vi "LED Main Loop.vi"(8 "error in (no error)":errorcluster, 9 "switch queue":refnum<queue>, 10 "switch notifier":refnum<notifier>, 11 "main gui queue":refnum<queue>) -> (0 "error out":errorcluster)   [LabVIEW 2020]
uses:
  GUI/Main GUI Loop/Handler.ctl
  Hardware/Actuators/Switches/Switch.lvclass
  C:/Users/jharw/Documents/1 Folder to Rule them All/UMD/Inflation-Apparatus/src/Hardware/General Hardware.lvclass
  Hardware/General Hardware.lvclass/General Hardware.ctl
  Hardware/Actuators/Switches/Switch.lvclass/Switch.ctl
  Hardware/General Hardware.lvclass
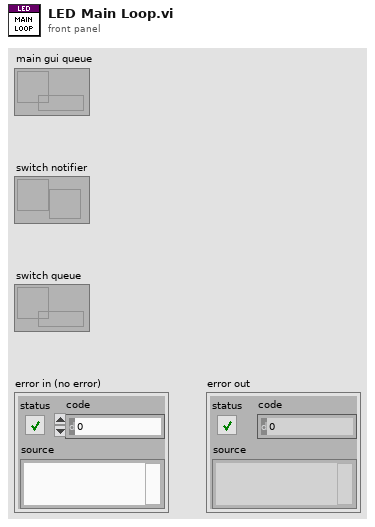
[diagram p1: front panel]
types:
  T1 = typedef "Handler.ctl" = cluster{"bool ref":refnum<vi>, "error":errorcluster, "msg":string, "status":string, "switch status":bool, "force cal":dbl[][], "force cal results":dbl[][]}
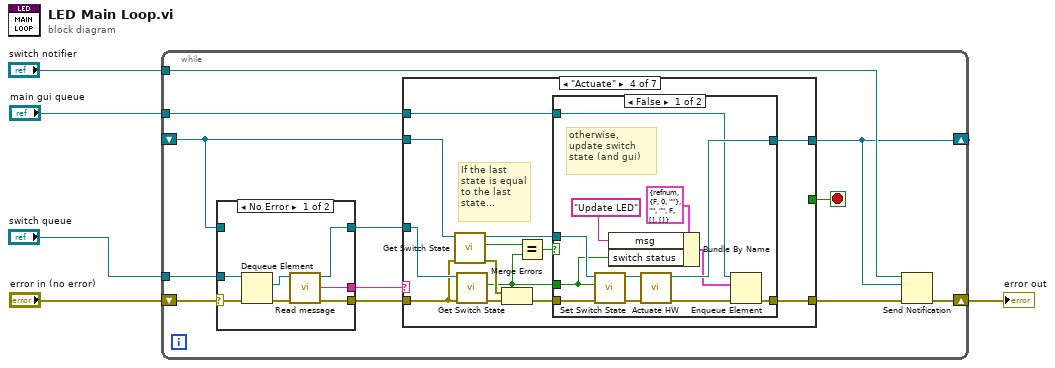
[diagram p0: block diagram]
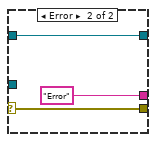
[diagram p2: hidden frame]
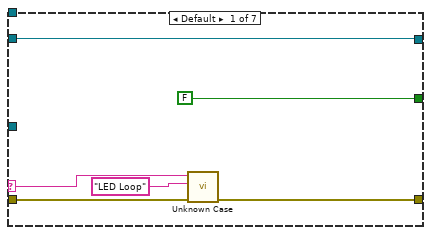
[diagram p3: hidden frame]
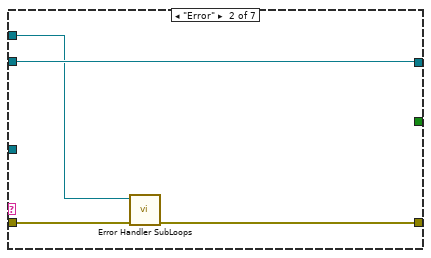
[diagram p4: hidden frame]
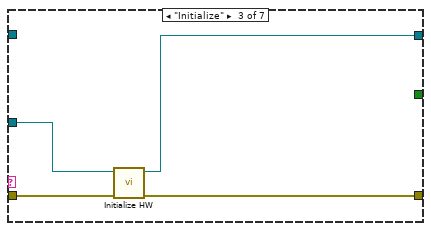
[diagram p5: hidden frame]
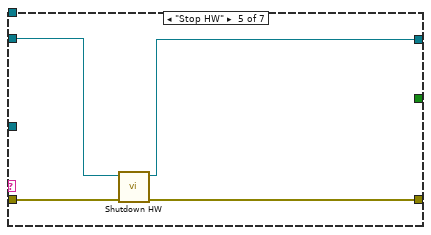
[diagram p7: hidden frame]
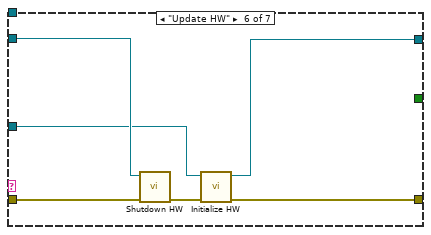
[diagram p8: hidden frame]
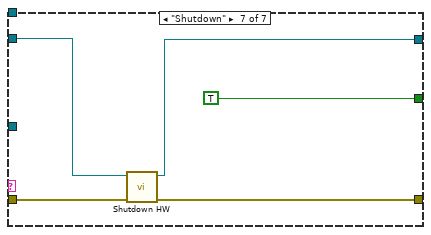
[diagram p9: hidden frame]
diagram:
  n1 = while {
    tunnel: "main gui queue" -> [w14]
    shift-right: [w8] -> w5
    shift-left: "error in (no error)" -> [w15]
    shift-right: [w6] -> _
    shift-left: _ -> [w12]
    tunnel: "switch queue" -> [w10]
    tunnel: "switch notifier" -> [w7]
    stop <- w11 stop-if-true
    n2 = case shown="No Error" w15 {
      selector: w15 -> [w18 w27]
      tunnel: [w24 w27] -> w17
      tunnel: [w22 "Error" ("message")] -> w16
      tunnel: [w23 w25] -> w13
      tunnel: w12 -> [_ w25]
      tunnel: w10 -> [w19 _]
      frame No Error {
        n3 = Dequeue Element(queue=w19, error in (no error)=w18) -> (element=w21:refnum<class "Switch.lvclass">, error out=w20:errorcluster)  [unwired: 1 in, 2 out]
        n4 = call "Read message.vi"("error in (no error)"=w20, "General Hardware in"=w21) -> ("error out"=w24:errorcluster, "message"=w22:string, "General Hardware out"=w23:refnum<class "Switch.lvclass">)  [unwired: 7 in]
      }
      frame Error {
      }
    }
    n5 = case shown="\"Actuate\"" w16 {
      selector: w16 -> [w31 _ _ _ _ _ _]
      tunnel: w17 -> [w33 w36 w41 w50 w72 w78 w82]
      tunnel: [w32 w35 w40 w53 w71 w76 w81] -> w9
      tunnel: w14 -> [_ w34 _ w42 _ _ _]
      tunnel: w13 -> [_ _ w38 w54 _ w74 _]
      tunnel: [w29 w37 w39 w52 w69 w73 w79] -> w6
      tunnel: w12 -> [w29 w37 _ w51 w70 w75 w80]
      tunnel: [FALSE _ _ _ _ _ TRUE] -> w11
      frame Default {
        n6 = call "Unknown Case.vi"("error in (no error)"=w33, "source"="LED Loop", "case"=w31) -> ("error out"=w32:errorcluster)  [unwired: 8 in]
      }
      frame "Error" {
        n7 = call "Error Handler SubLoops.vi"("error in"=w36, "main gui queue"=w34) -> ("error out"=w35:errorcluster)  [unwired: 9 in]
      }
      frame "Initialize" {
        n8 = call-dynamic "Initialize HW.vi"("error in (no error)"=w41, "Switch in"=w38) -> ("error out"=w40:errorcluster, "Switch out"=w39:refnum<class "Switch.lvclass">)  [unwired: 8 in]
      }
      frame "Actuate" {
        # "If the last state is equal to the last state..."
        n9 = call "Get Switch State.vi"("error in (no error)"=w50, "Switch in"=w51) -> ("error out"=w47:errorcluster, "switch state"=w45:bool, "Switch out"=w46:refnum<class "Switch.lvclass">)  [unwired: 7 in]
        n10 = call "Get Switch State.vi"("error in (no error)"=w50, "Switch in"=w54) -> ("error out"=w48:errorcluster, "switch state"=w44:bool)  [unwired: 7 in, 1 out]
        n11 = Merge Errors(w47, w48) -> (w49:errorcluster)
        n12 = Equal?(x=w45, y=w44) -> (x = y?=w43:bool)
        n13 = case shown="False" w43 {
          tunnel: [w60 w68] -> w53
          tunnel: [w64 w67] -> w52
          tunnel: w49 -> [w63 w68]
          tunnel: w46 -> [w62 w67]
          tunnel: w44 -> [w56 _]
          tunnel: w42 -> [w59 _]
          frame False {
            # "otherwise, update switch state (and gui)"
            n14 = call "Set Switch State.vi"("error in (no error)"=w63, "switch state"=w56, "Switch in"=w62) -> ("error out"=w65:errorcluster, "Switch out"=w66:refnum<class "Switch.lvclass">)  [unwired: 7 in]
            n15 = Bundle By Name(cluster=T1 {"bool ref"=refnum, "error"={"status"=FALSE, "code"=0, "source"=""}, "msg"="", "status"="", "switch status"=FALSE, "force cal"=[], "force cal results"=[]} ("element"), "msg"="Update LED", "switch status"=w56) -> (w57:T1)
            n16 = call-dynamic "Actuate HW.vi"("error in (no error)"=w65, "Switch in"=w66) -> ("error out"=w61:errorcluster, "Switch out"=w64:refnum<class "Switch.lvclass">)  [unwired: 8 in]
            n17 = Enqueue Element(queue=w59, element=w57, error in (no error)=w61) -> (error out=w60:errorcluster)  [unwired: 1 in, 2 out]
          }
          frame True {
            # "do nothing"
          }
        }
      }
      frame "Stop HW" {
        n18 = call-dynamic "Shutdown HW.vi"("error in (no error)"=w72, "Switch in"=w70) -> ("error out"=w71:errorcluster, "Switch out"=w69:refnum<class "Switch.lvclass">)  [unwired: 8 in]
      }
      frame "Update HW" {
        n19 = call-dynamic "Shutdown HW.vi"("error in (no error)"=w78, "Switch in"=w75) -> ("error out"=w77:errorcluster)  [unwired: 8 in, 1 out]
        n20 = call-dynamic "Initialize HW.vi"("error in (no error)"=w77, "Switch in"=w74) -> ("error out"=w76:errorcluster, "Switch out"=w73:refnum<class "Switch.lvclass">)  [unwired: 8 in]
      }
      frame "Shutdown" {
        n21 = call-dynamic "Shutdown HW.vi"("error in (no error)"=w82, "Switch in"=w80) -> ("error out"=w81:errorcluster, "Switch out"=w79:refnum<class "Switch.lvclass">)  [unwired: 8 in]
      }
    }
    n22 = Send Notification(notification=w6, notifier=w7, error in (no error)=w9) -> (error out=w8:errorcluster)  [unwired: 1 out]
  }
  "error out" <- w5
